vi "List Objects.vi"(8 "error in (no error)":errorcluster, 9 "Prefix":string, 10 "Delimiter":string, 11 "Bucket in":refnum<class "Bucket.lvclass">) -> (0 "error out":errorcluster, 2 "Objects":T1[](array[typedef]), 3 "Bucket out":refnum<class "Bucket.lvclass">)   [LabVIEW 2015, in "NI_AWS_S3.lvlib" / "Bucket.lvclass"]
uses:
  Bucket.lvclass
  Object/Object.lvclass
  Object Content.ctl
  Storage Class.ctl
  Owner.ctl
  Core/HTTP Request/Request Options.ctl
  Core/HTTP Request/Name Value Pair.ctl
  Core/HTTP Request/Region handling.ctl
  Core/HTTP Request/URL formatting.ctl
  Bucket.lvclass/Bucket.ctl
  Read Name.vi
  Core/HTTP Request/HTTP Request.lvclass
  NI_AWS_S3.lvlib
panel:
  out "Objects":refnum<class "Object.lvclass">[](array[class])
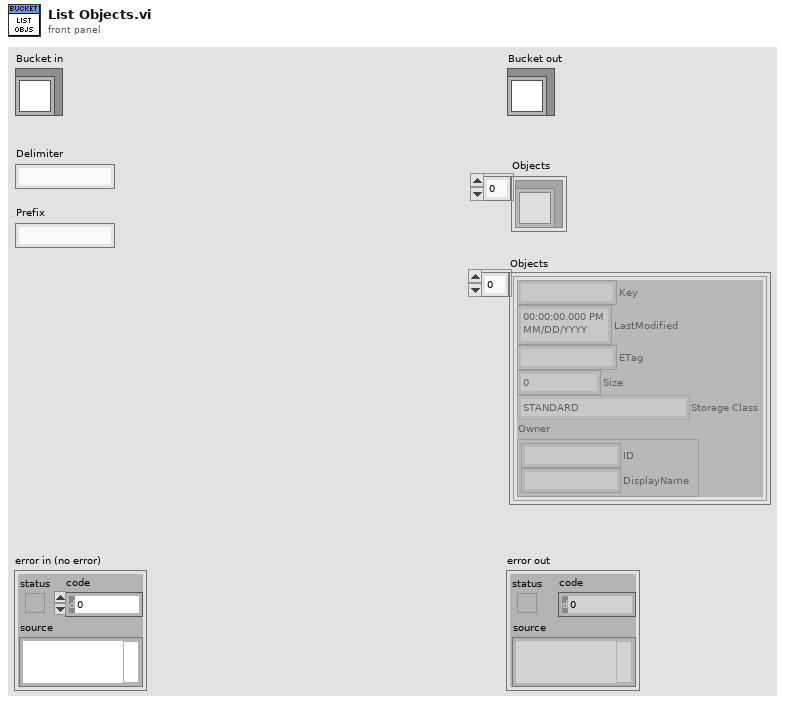
[diagram p1: front panel]
types:
  T1 = typedef "NI_AWS_S3.lvlib/Object Content.ctl" = cluster{"Key":string, "LastModified":timestamp, "ETag":string, "Size":u64, "Storage Class":T2, "Owner":T3}
  T2 = typedef "NI_AWS_S3.lvlib/Storage Class.ctl" = enum16{"STANDARD", "REDUCED_REDUNDANCY"}
  T3 = typedef "NI_AWS_S3.lvlib/Owner.ctl" = cluster{"ID":string, "DisplayName":string}
  T4 = typedef "NI_AWS_Core.lvlib/HTTP Request.lvclass/Name Value Pair.ctl" = cluster{"name":string, "value":string}
  T5 = typedef "NI_AWS_Core.lvlib/HTTP Request.lvclass/Region handling.ctl" = enum16{"use region everywhere", "use region (authentication only)", "use region (URL only)", "ignore region everwhere"}
  T6 = typedef "NI_AWS_Core.lvlib/HTTP Request.lvclass/Request Options.ctl" = cluster{"request headers":T4[], "request parameters":T4[], "request body":string, "region handling":T5, "URL formatting":T7}
  T7 = typedef "NI_AWS_Core.lvlib/HTTP Request.lvclass/URL formatting.ctl" = enum16{"region-", "region."}
  T8 = typedef "NI_AWS_Core.lvlib/HTTP Request.lvclass/Response.ctl" = cluster{"Headers":string, "Body":string}
  T9 = typedef "NI_AWS_S3.lvlib/List Objects Result.ctl" = cluster{"Name":string, "Prefix":string, "Marker":string, "MaxKeys":u16, "IsTruncated?":bool, "Contents":T1[], "CommonPrefixes":T10[]}
  T10 = typedef "NI_AWS_S3.lvlib/Common Prefix.ctl" = cluster{"Prefix":string}
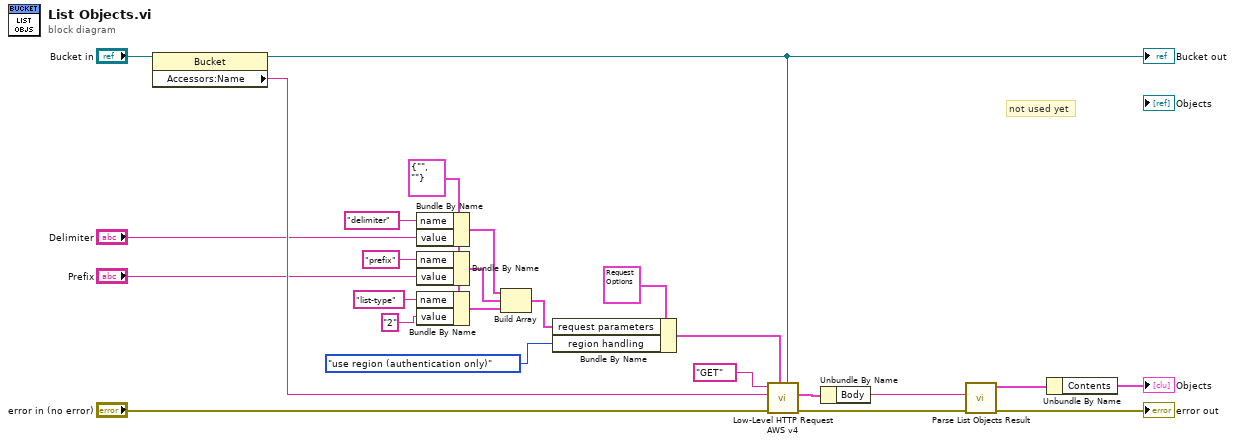
[diagram p0: block diagram]
diagram:
  w7 = T4 {"name"="", "value"=""} ("Name Value Pair")
  # "not used yet"
  n1 = property class="Bucket"(reference="Bucket in") -> (reference out=w20:refnum<class "Bucket.lvclass">, "Accessors:Name"=w19:string)  [unwired: 1 in, 1 out]
  "Bucket out" <- w20
  n2 = Bundle By Name(cluster=w7, "name"="delimiter", "value"="Delimiter") -> (w8:T4)
  n3 = Bundle By Name(cluster=w7, "name"="prefix", "value"="Prefix") -> (w9:T4)
  n4 = Bundle By Name(cluster=w7, "name"="list-type", "value"="2") -> (w15:T4)
  n5 = Build Array(w8, w9, w15) -> (w14:T4[])
  n6 = Bundle By Name(cluster=T6 {"request headers"=[], "request parameters"=[], "request body"="", "region handling"=enum."use region everywhere", "URL formatting"=enum."region."} ("Request Options"), "request parameters"=w14, "region handling"=Region_handling."use region (authentication only)") -> (w22:T6)
  n7 = call "Low-Level HTTP Request AWS v4.vi"("AWS Core"=w20, "Request Options"=w22, "error in (no error)"="error in (no error)", "URL Prefix"=w19, "HTTP-Verb"="GET") -> ("error out"=w4:errorcluster, "Response"=w6:T8)  [unwired: 4 in, 1 out]
  n8 = Unbundle By Name(w6) -> ("Body"=w5:string)
  n9 = call "Parse List Objects Result.vi"("error in (no error)"=w4, "Response body"=w5) -> ("error out"=→"error out":errorcluster, "List Objects Result"=w2:T9)  [unwired: 8 in]
  n10 = Unbundle By Name(w2) -> ("Contents"=→"Objects":T1[])
